vi "Queue growth test.vi"() -> ()   [LabVIEW 2024]
panel:
  in  "Repeat times":i32=1000000 format="%.0p"
  in  "max queue size (-1, unlimited)":i32=10 format="%.0p"
  out "overflow element":dbl[](array[numeric])
  in  "dimension size":i32=100 format="%.0p"
  out "created new?":bool
  out "overflow?":bool
  out "max queue size":i32
  out "queue name":string
  out "# pending remove":i32
  out "# pending insert":i32
  out "# elements in queue":i32
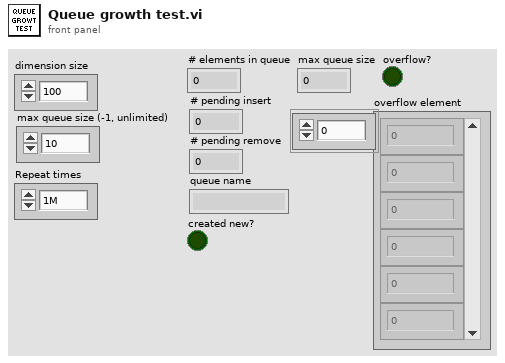
[diagram p1: front panel]
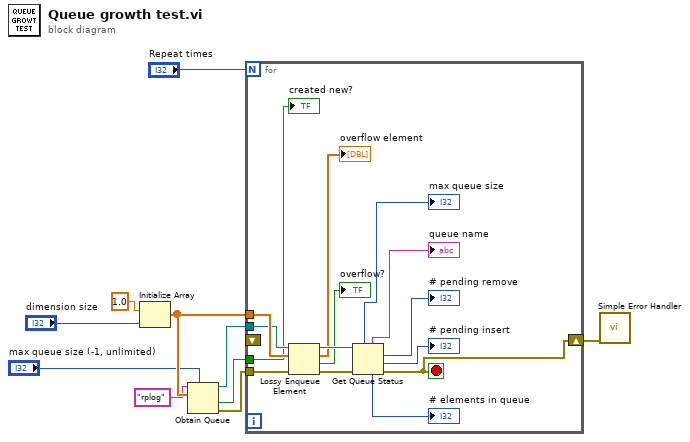
[diagram p0: block diagram]
diagram:
  n1 = Initialize Array(1.0 ("element"), "dimension size") -> (w8:dbl[])
  n2 = Obtain Queue(max queue size (-1, unlimited)="max queue size (-1, unlimited)", name (unnamed)="rplog", element data type=w8) -> (queue out=w3:refnum<queue>, created new?=w2:bool, error out=w1:errorcluster)  [unwired: 2 in]
  n3 = for {
    N: "Repeat times" -> [_]
    tunnel: w8 -> [w16]
    shift-right: [w15] -> w7
    shift-left: _ -> [_]
    tunnel: w3 -> [w13]
    tunnel: w2 -> [w12]
    tunnel: w1 -> [w11]
    stop <- w15 stop-if-true
    n4 = Lossy Enqueue Element(queue=w13, element=w16, error in (no error)=w11) -> (queue out=w18:refnum<queue>, overflow element=→"overflow element":dbl[], overflow?=→"overflow?":bool, error out=w19:errorcluster)
    n5 = Get Queue Status(queue=w18, error in (no error)=w19) -> (queue name=→"queue name":string, max queue size=→"max queue size":i32, # pending remove=→"# pending remove":i32, # pending insert=→"# pending insert":i32, error out=w15:errorcluster, # elements in queue=→"# elements in queue":i32)  [unwired: 1 in, 2 out]
    "created new?" <- w12
  }
  n6 = call <vilib>:"Simple Error Handler.vi"("error in (no error)"=w7) -> ()  [unwired: 4 in, 5 out]
